vi "csv_control _02.vi"() -> (3 "pass":bool)   [LabVIEW 2024]
panel:
  in  "错误输入":errorcluster
  out "错误输出":errorcluster
  in  "Test_Value":dbl
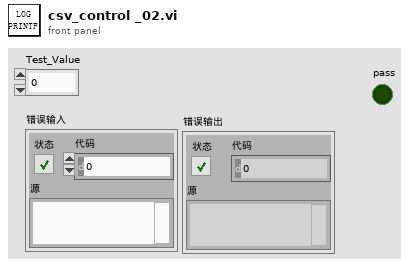
[diagram p1: front panel]
types:
  T1 = enum16{"open", "replace", "create", "open or create", "replace or create", "replace or create with confirmation"}
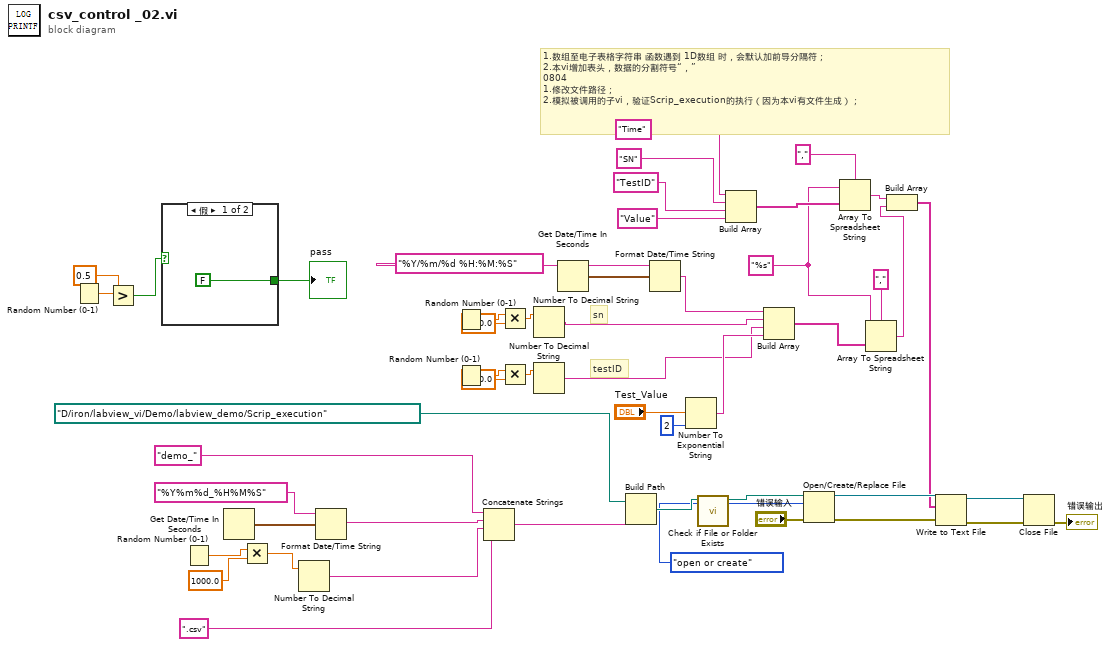
[diagram p0: block diagram]
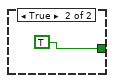
[diagram p2: hidden frame]
diagram:
  w26 = "%s" ("格式字符串")
  # "testID"
  # "sn"
  # "1.数组至电子表格字符串 函数遇到 1D数组 时，会默认加前导分隔符；\n2.本vi增加表头，数据的分割符号“，”\n0804\n1.修改文件路径；\n2.模拟被调用的子vi，验证Scrip_execution的执行（因为本vi有文件生成）；"
  n1 = Random Number (0-1)() -> (number: 0 to 1=w9:dbl)
  n2 = Greater?(x=w9, y=0.5) -> (0:w6:bool)
  n3 = case shown="假" w6 {
    tunnel: [FALSE TRUE] -> w7
    frame False {
    }
    frame True {
    }
  }
  "pass" <- w7
  n4 = Random Number (0-1)() -> (number: 0 to 1=w5:dbl)
  n5 = Get Date/Time In Seconds() -> (seconds since 1Jan1904=w35:timestamp)
  n6 = Multiply(x=w5, y=1000.0) -> (x*y=w3:dbl)
  n7 = Number To Decimal String(number=w3) -> (decimal integer string=w2:string)  [unwired: 1 in]
  n8 = Format Date/Time String(time format string (%c)="%Y%m%d_%H%M%S" ("时间格式字符串(%c)"), seconds (now)=w35) -> (date/time string=w34:string)  [unwired: 1 in]
  n9 = Random Number (0-1)() -> (number: 0 to 1=w21:dbl)
  n10 = Random Number (0-1)() -> (number: 0 to 1=w15:dbl)
  n11 = Concatenate Strings("demo_" ("字符串"), w34, w2, ".csv" ("字符串")) -> (w37:string)
  n12 = Multiply(x=w21, y=1000.0) -> (x*y=w19:dbl)
  n13 = Multiply(x=w15, y=1000.0) -> (x*y=w17:dbl)
  n14 = Number To Decimal String(number=w19) -> (decimal integer string=w18:string)  [unwired: 1 in]
  n15 = Number To Decimal String(number=w17) -> (decimal integer string=w14:string)  [unwired: 1 in]
  n16 = Get Date/Time In Seconds() -> (seconds since 1Jan1904=w46:timestamp)
  n17 = Build Path(base path=path "D:/iron/labview_vi/Demo/labview_demo/Scrip_execution" ("基路径"), name or relative path=w37) -> (appended path=w50:path)
  n18 = Format Date/Time String(time format string (%c)="%Y/%m/%d %H:%M:%S" ("时间格式字符串(%c)"), seconds (now)=w46) -> (date/time string=w33:string)  [unwired: 1 in]
  n19 = Number To Exponential String(number="Test_Value", precision (6)=i16 2 ("精度(6)")) -> (E-format string=w47:string)  [unwired: 2 in]
  n20 = call <vilib>:"Check if File or Folder Exists.vi"("path"=w50) -> ("dup path"=w49:path)  [unwired: 8 in, 2 out]
  n21 = Build Array("Time" ("元素"), "SN" ("元素"), "TestID" ("元素"), "Value" ("元素")) -> (w27:string[])
  n22 = Build Array(w33, w18, w14, w47) -> (w44:string[])
  n23 = Open/Create/Replace File(file path (use dialog)=w49, error in="错误输入", operation (0:open)=T1."open or create" ("操作(0:open)")) -> (refnum out=w42:refnum<file>, error out=w13:errorcluster)  [unwired: 3 in, 1 out]
  n24 = Array To Spreadsheet String(delimiter (Tab)="," ("分隔符(Tab)"), array=w27, 3:w26) -> (spreadsheet string=w24:string)
  n25 = Array To Spreadsheet String(delimiter (Tab)="," ("分隔符(Tab)"), array=w44, 3:w26) -> (spreadsheet string=w23:string)
  n26 = Build Array(w24, w23) -> (w22:string[])
  n27 = Write to Text File(file (use dialog)=w42, text=w22, error in=w13) -> (refnum out=w41:refnum<file>, error out=w12:errorcluster)  [unwired: 1 in, 1 out]
  n28 = Close File(refnum=w41, error in=w12) -> (error out=→"错误输出":errorcluster)  [unwired: 1 out]
